vi "MCA.vi"(0 "Velocity":cluster{"vx":dbl, "vy":dbl, "vy":dbl}, 1 "xlp":dbl=0.1 caption="Pitch A Gain", 2 "xhp":dbl=0.001 caption="Pitch V Gain", 5 "Acceleration":cluster{"ax":dbl, "ay":dbl, "az":dbl}, 7 "xrl":dbl=10.0 caption="Pitch Tilt limit", 9 "yrl":dbl=10.0 caption="Roll Tilt limit", 11 "zl":dbl=0.01 caption="Heave limit", 12 "ylp":dbl=0.08 caption="Roll A Gain", 13 "yhp":dbl=0.0008 caption="Roll V Gain", 14 "zhp":dbl=0.05 caption="Heave Gain") -> (4 "Rotations":cluster{"Pitch":dbl, "Roll":dbl, "yaw ":dbl}, 15 "Heave":dbl)   [LabVIEW 2019]
uses:
  <vilib>/Analysis/3filter.llb/Filter Passband Type.ctl
  <vilib>/ptbypt/NI_PtbyPt.lvlib
  <vilib>/Analysis/NI_AALBase.lvlib
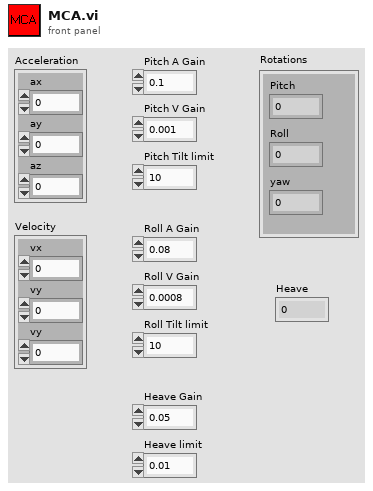
[diagram p1: front panel]
types:
  T1 = typedef "NI_AALBase.lvlib/Filter Passband Type.ctl" = enum32{"Lowpass", "Highpass", "Bandpass", "Bandstop"}
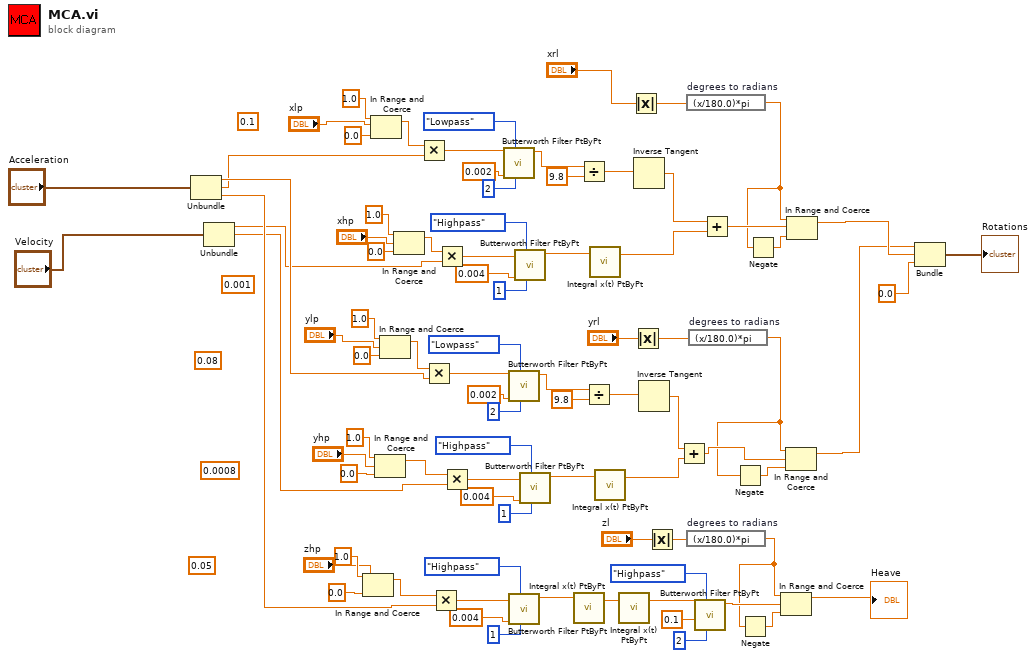
[diagram p0: block diagram]
diagram:
  (unwired) 0.05 ("x")
  (unwired) 0.0008 ("x")
  (unwired) 0.08 ("x")
  (unwired) 0.001 ("x")
  (unwired) 0.1 ("x")
  n1 = Unbundle("Acceleration") -> ("ax"=w6:dbl, "ay"=w5:dbl, "az"=w19:dbl)
  n2 = Unbundle("Velocity") -> ("vx"=w3:dbl, "vy"=w4:dbl)  [unwired: 1 out]
  n3 = In Range and Coerce(upper limit=1.0, x="zhp", lower limit=0.0) -> (coerced(x)=w21:dbl)  [unwired: 1 out]
  n4 = In Range and Coerce(upper limit=1.0, x="xlp", lower limit=0.0) -> (coerced(x)=w37:dbl)  [unwired: 1 out]
  n5 = In Range and Coerce(upper limit=1.0, x="yhp", lower limit=0.0) -> (coerced(x)=w46:dbl)  [unwired: 1 out]
  n6 = In Range and Coerce(upper limit=1.0, x="ylp", lower limit=0.0) -> (coerced(x)=w49:dbl)  [unwired: 1 out]
  n7 = In Range and Coerce(upper limit=1.0, x="xhp", lower limit=0.0) -> (coerced(x)=w41:dbl)  [unwired: 1 out]
  n8 = Multiply(x=w37, y=w5) -> (x*y=w75:dbl)
  n9 = Multiply(x=w49, y=w6) -> (x*y=w58:dbl)
  n10 = Multiply(x=w21, y=w19) -> (x*y=w33:dbl)
  n11 = Multiply(x=w41, y=w3) -> (x*y=w76:dbl)
  n12 = Multiply(x=w46, y=w4) -> (x*y=w59:dbl)
  n13 = call <vilib>:"Butterworth Filter PtByPt.vi"("order"=2, "filter type"=Filter_Passband_Type."Lowpass", "low cutoff freq: fl"=0.002, "x"=w75) -> ("Filtered x"=w73:dbl)  [unwired: 5 in, 1 out]
  n14 = call <vilib>:"Butterworth Filter PtByPt.vi"("order"=2, "filter type"=Filter_Passband_Type."Lowpass", "low cutoff freq: fl"=0.002, "x"=w58) -> ("Filtered x"=w56:dbl)  [unwired: 5 in, 1 out]
  n15 = call <vilib>:"Butterworth Filter PtByPt.vi"("order"=1, "filter type"=Filter_Passband_Type."Highpass", "low cutoff freq: fl"=0.004, "x"=w33) -> ("Filtered x"=w28:dbl)  [unwired: 5 in, 1 out]
  n16 = call <vilib>:"Butterworth Filter PtByPt.vi"("order"=1, "filter type"=Filter_Passband_Type."Highpass", "low cutoff freq: fl"=0.004, "x"=w76) -> ("Filtered x"=w71:dbl)  [unwired: 5 in, 1 out]
  n17 = call <vilib>:"Butterworth Filter PtByPt.vi"("order"=1, "filter type"=Filter_Passband_Type."Highpass", "low cutoff freq: fl"=0.004, "x"=w59) -> ("Filtered x"=w54:dbl)  [unwired: 5 in, 1 out]
  n18 = call <vilib>:"Integral x(t) PtByPt.vi"("x"=w28) -> ("integral x(t)"=w27:dbl)  [unwired: 3 in, 1 out]
  n19 = Divide(x=w73, y=9.8) -> (x/y=w74:dbl)
  n20 = Divide(x=w56, y=9.8) -> (x/y=w57:dbl)
  n21 = call <vilib>:"Integral x(t) PtByPt.vi"("x"=w71) -> ("integral x(t)"=w70:dbl)  [unwired: 3 in, 1 out]
  n22 = call <vilib>:"Integral x(t) PtByPt.vi"("x"=w54) -> ("integral x(t)"=w53:dbl)  [unwired: 3 in, 1 out]
  n23 = call <vilib>:"Integral x(t) PtByPt.vi"("x"=w27) -> ("integral x(t)"=w29:dbl)  [unwired: 3 in, 1 out]
  n24 = Absolute Value(x="xrl") -> (abs(x)=w68:dbl)
  n25 = Absolute Value(x="yrl") -> (abs(x)=w35:dbl)
  n26 = Inverse Tangent(1:w74) -> (0:w72:dbl)
  n27 = Inverse Tangent(1:w57) -> (0:w55:dbl)
  n28 = Absolute Value(x="zl") -> (abs(x)=w17:dbl)
  n29 = Add(x=w55, y=w53) -> (x+y=w36:dbl)
  n30 = expression code="(x/180.0)*pi" "degrees to radians"(w68) -> (w12:dbl)
  n31 = expression code="(x/180.0)*pi" "degrees to radians"(w17) -> (w10:dbl)
  n32 = expression code="(x/180.0)*pi" "degrees to radians"(w35) -> (w14:dbl)
  n33 = call <vilib>:"Butterworth Filter PtByPt.vi"("order"=2, "filter type"=Filter_Passband_Type."Highpass", "high cutoff freq: fh"=0.1, "x"=w29) -> ("Filtered x"=w18:dbl)  [unwired: 5 in, 1 out]
  n34 = Add(x=w72, y=w70) -> (x+y=w69:dbl)
  n35 = Negate(x=w14) -> (-x=w15:dbl)
  n36 = Negate(x=w10) -> (-x=w11:dbl)
  n37 = Negate(x=w12) -> (-x=w13:dbl)
  n38 = In Range and Coerce(upper limit=w10, x=w18, lower limit=w11) -> (coerced(x)=→"Heave":dbl)  [unwired: 1 out]
  n39 = In Range and Coerce(upper limit=w14, x=w36, lower limit=w15) -> (coerced(x)=w1:dbl)  [unwired: 1 out]
  n40 = In Range and Coerce(upper limit=w12, x=w69, lower limit=w13) -> (coerced(x)=w2:dbl)  [unwired: 1 out]
  n41 = Bundle(w1, w2, "Numeric"=0.0) -> (→"Rotations":cluster{dbl, dbl, "Numeric":dbl})  [unwired: 1 in]
